vi "Adquirir Imagen.vi"(8 "error in (no error)":errorcluster, 11 "Webcam in":refnum<class "Webcam.lvclass">) -> (0 "error out":errorcluster, 2 "Imagen":T1, 3 "Webcam out":refnum<class "Webcam.lvclass">)   [LabVIEW 2020, in "Webcam.lvclass"]
uses:
  Webcam.lvclass
  C:/Users/enoea/Desktop/DemoOOP/Clases/Abstracta/Camara/Camara.lvclass
  <vilib>/vision/Image Controls.llb/IMAQ Image.ctl
  Webcam.lvclass/Webcam.ctl
  Abstracta/Camara/Camara.lvclass/Camara.ctl
  Read Session Out.vi
  Abstracta/Camara/Read New Image.vi
  <vilib>/vision/driver/NI_Vision_Acquisition_Software.lvlib
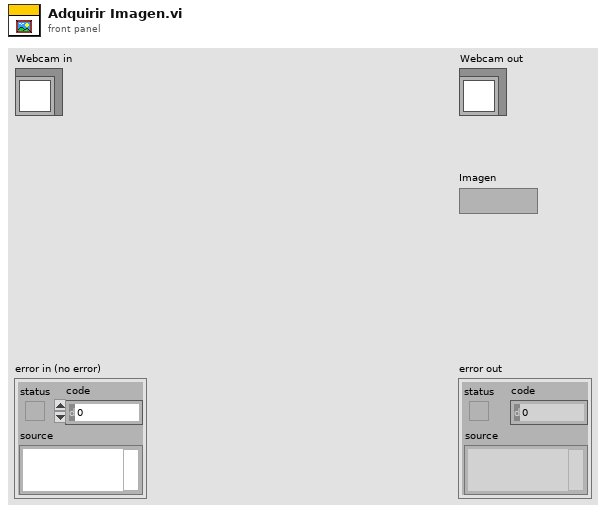
[diagram p1: front panel]
types:
  T1 = typedef "IMAQ Image.ctl" = refnum<image>
  T2 = typedef "IMAQdx.ctl" = refnum<k21>
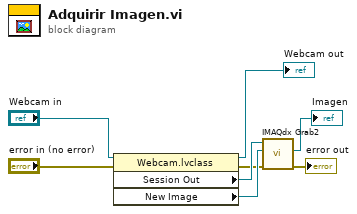
[diagram p0: block diagram]
diagram:
  n1 = property class="Webcam.lvclass"(reference="Webcam in", error in="error in (no error)") -> (reference out=→"Webcam out":refnum<class "Webcam.lvclass">, error out=w2:errorcluster, "Session Out"=w4:T2, "New Image"=w3:T1)
  n2 = call <vilib>:"IMAQdx Grab2.vi"("error in"=w2, "Image In"=w3, "Session In"=w4) -> ("error out"=→"error out":errorcluster, "Image Out"=→"Imagen":T1)  [unwired: 5 in, 2 out]
